vi "Weighted Mean_PN.vi"(2 "weights":dbl[](array[numeric]), 3 "1D data":dbl[](array[numeric])) -> (1 "Weighted mean":dbl)   [LabVIEW 2011]
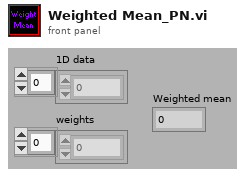
[diagram p1: front panel]
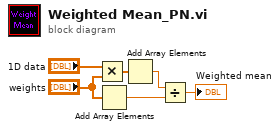
[diagram p0: block diagram]
diagram:
  n1 = Multiply(x="1D data", y="weights") -> (x*y=w6:dbl[])
  n2 = Add Array Elements(numeric array="weights") -> (sum=w2:dbl)
  n3 = Add Array Elements(numeric array=w6) -> (sum=w5:dbl)
  n4 = Divide(x=w5, y=w2) -> (x/y=→"Weighted mean":dbl)
